vi "DialogCloneMethod.vi"(0 "ClassWriterNative.lvclass":refnum<class "ClassWriterNative.lvclass">, 1 "VIItemRefIn":refnum<vi>, 5 "error in (no error)":errorcluster) -> (11 "NewVIDescriptionOut":string caption="New VI Description", 13 "OpenAfter":bool, 14 "ClassWriterGOOP300.lvclassOut":refnum<class "ClassWriterNative.lvclass">, 15 "VIItemRefOut":refnum<vi>, 16 "NewVIPath":path, 17 "Cancelled":bool, 18 "LibraryOwners":refnum<vi>[](array[refnum]), 19 "error out":errorcluster)   [LabVIEW 2020, in "ClassWriterNative.lvclass"]
uses:
  <resource>/Framework/Providers/Open_GDS/ClassProviders/Provider_LvNativeClass/ClassWriterNative_class/ClassWriterNative.lvclass
  <vilib>/Utility/lvfile.llb/NI_FileType.lvlib
panel:
  in  "Help":bool
  out "ProductPicture":picture
  in  "_NewVIDescription":string caption="New VI Description"
  in  "_CreateOpenVI":bool
  in  "_OverwirteTragetVIs":bool
  in  "_CloneMethodClasses":i32[](listbox) caption="Select which classes to clone the VI to"
  out "_ViPathAlreadyExists":bool=TRUE caption="This VI already exists"
  out "_CloneViName":string caption="Original VI Name"
  in  "_ClassOwner":u16(ring) caption="New VI Owner" items=["<No owner selected>", "<Clone VI to Selected Classes>"]
  in  "_ShowContextHelp":bool
  in  "_NewVIPath":path caption="New VI path"
  in  "_NewVIName":string caption="New VI name"
  in  "_Cancel":bool
  in  "_CloneVI":bool
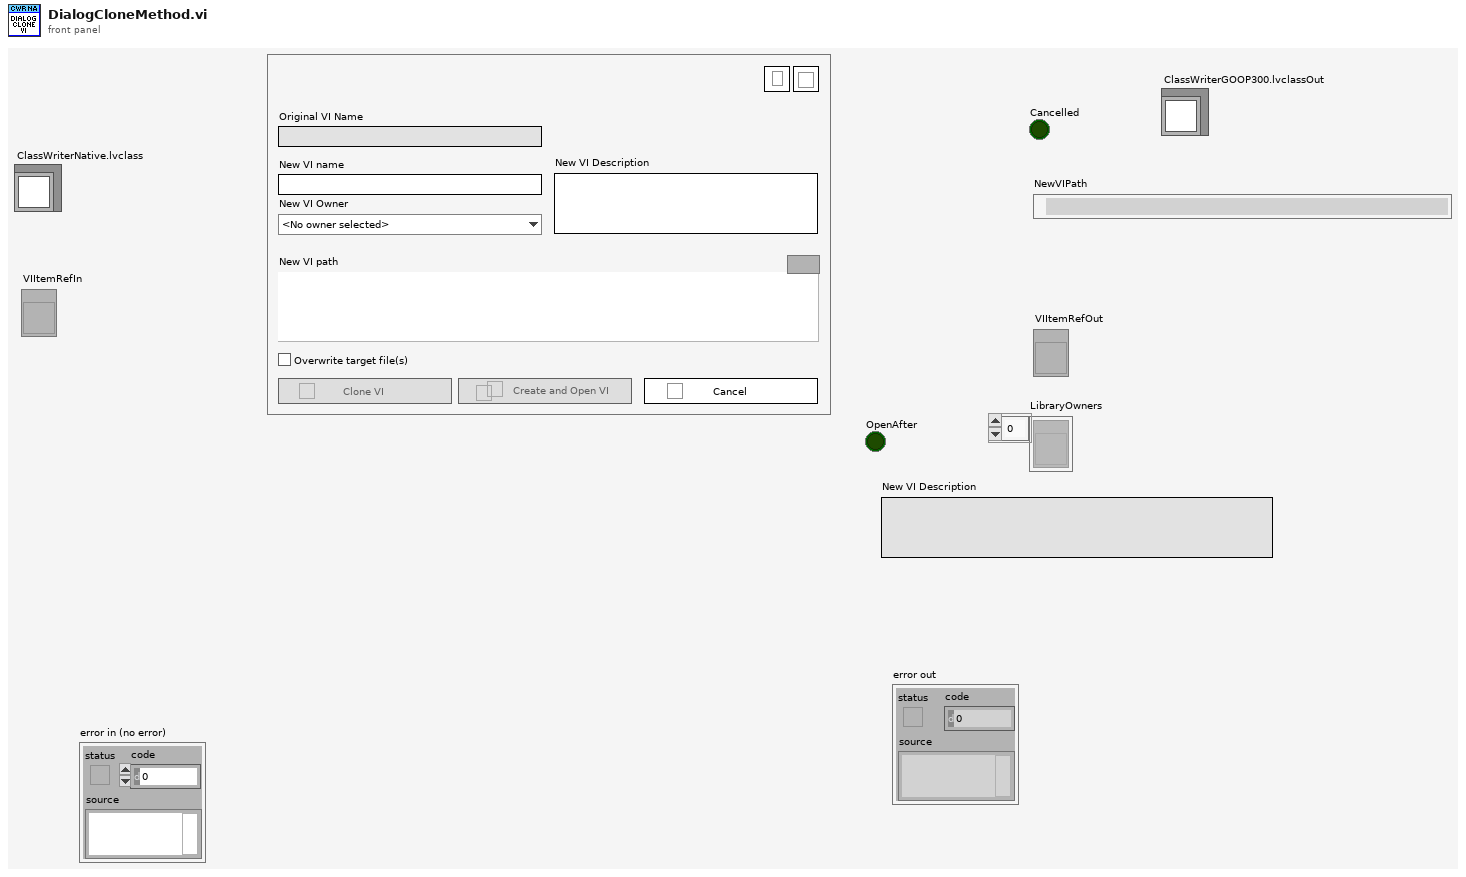
[diagram p1: front panel]
types:
  T1 = cluster{"Cancel":bool, "OrgVIPath":path, "VIName":string, "Libs":refnum<vi>[], "SiblingClasses":refnum<vi>[], "ProjectFolder":path, "ViRelFromParent":path, "VIExt":string, "ManyClasses":bool, "OrgLibName":string, "AllClasses":refnum<vi>[], "OpenAfter":bool}
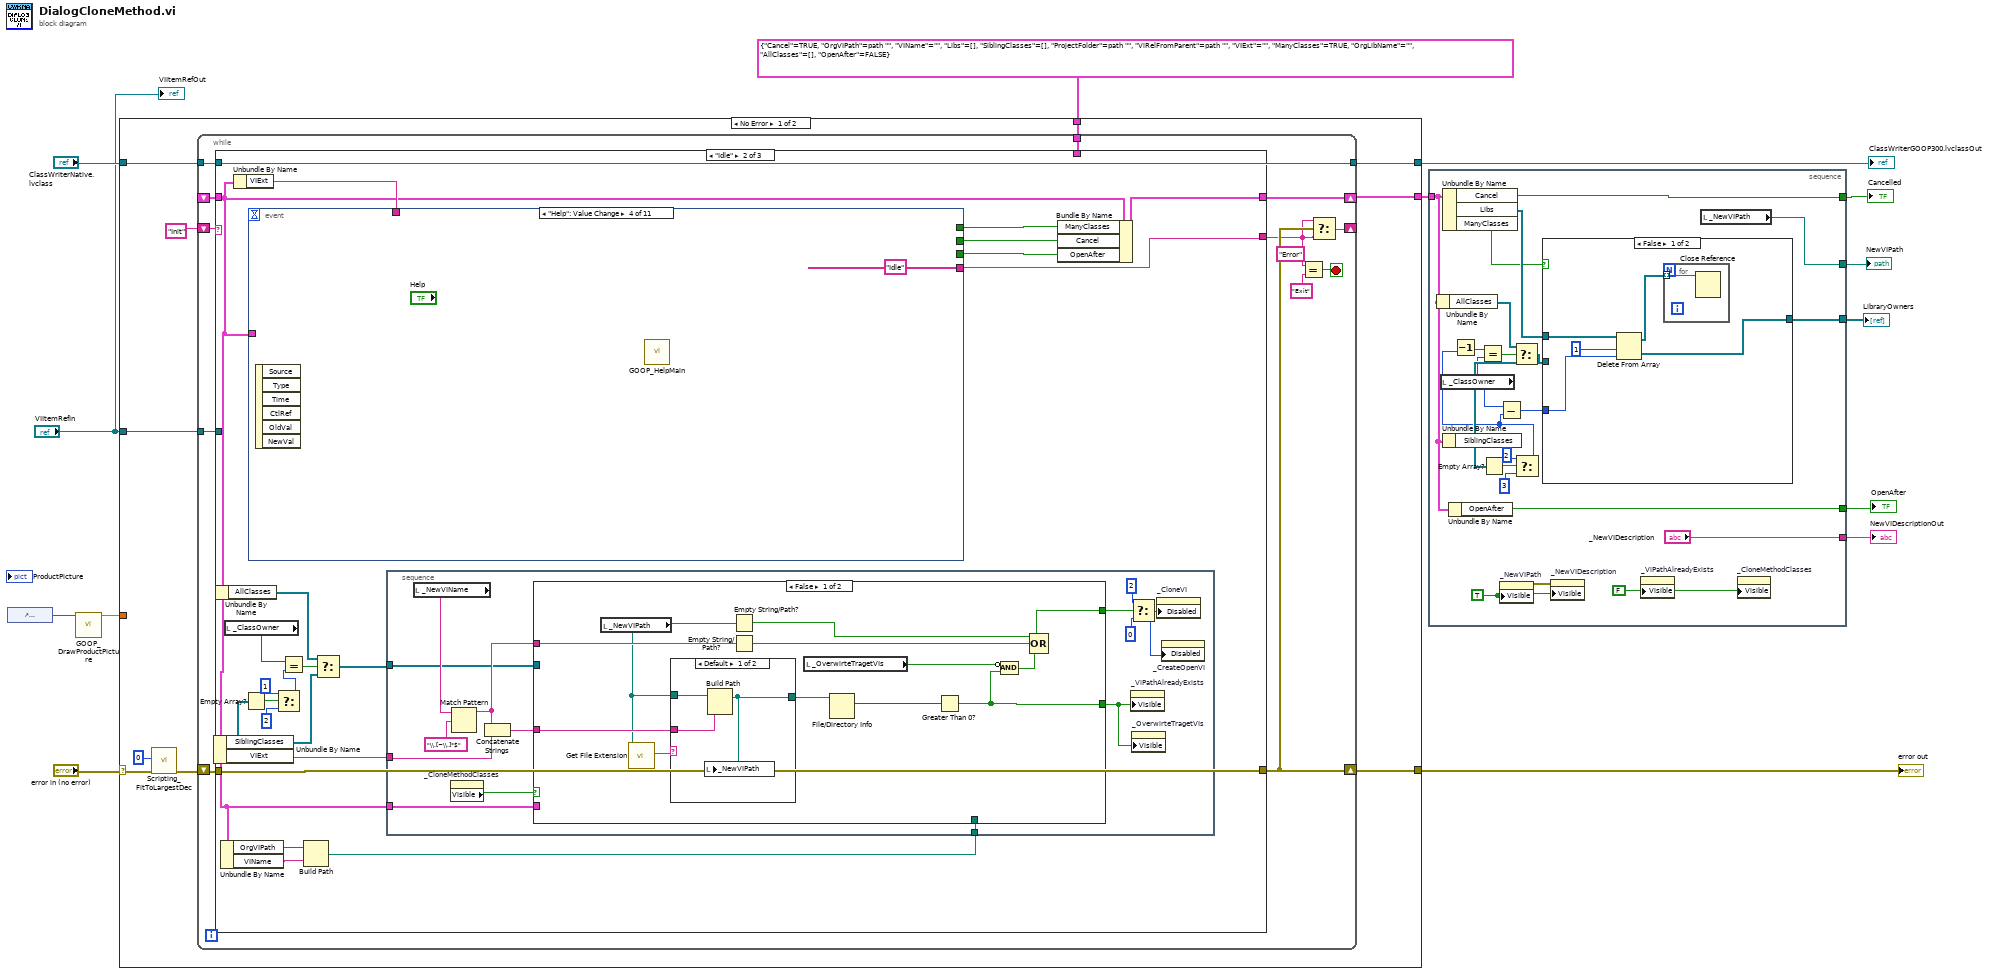
[diagram p0: block diagram]
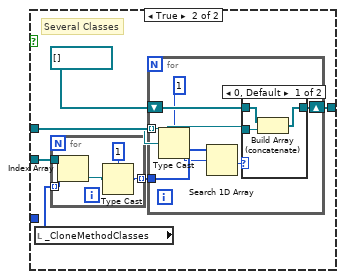
[diagram p2: hidden frame]
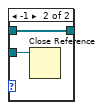
[diagram p3: hidden frame]
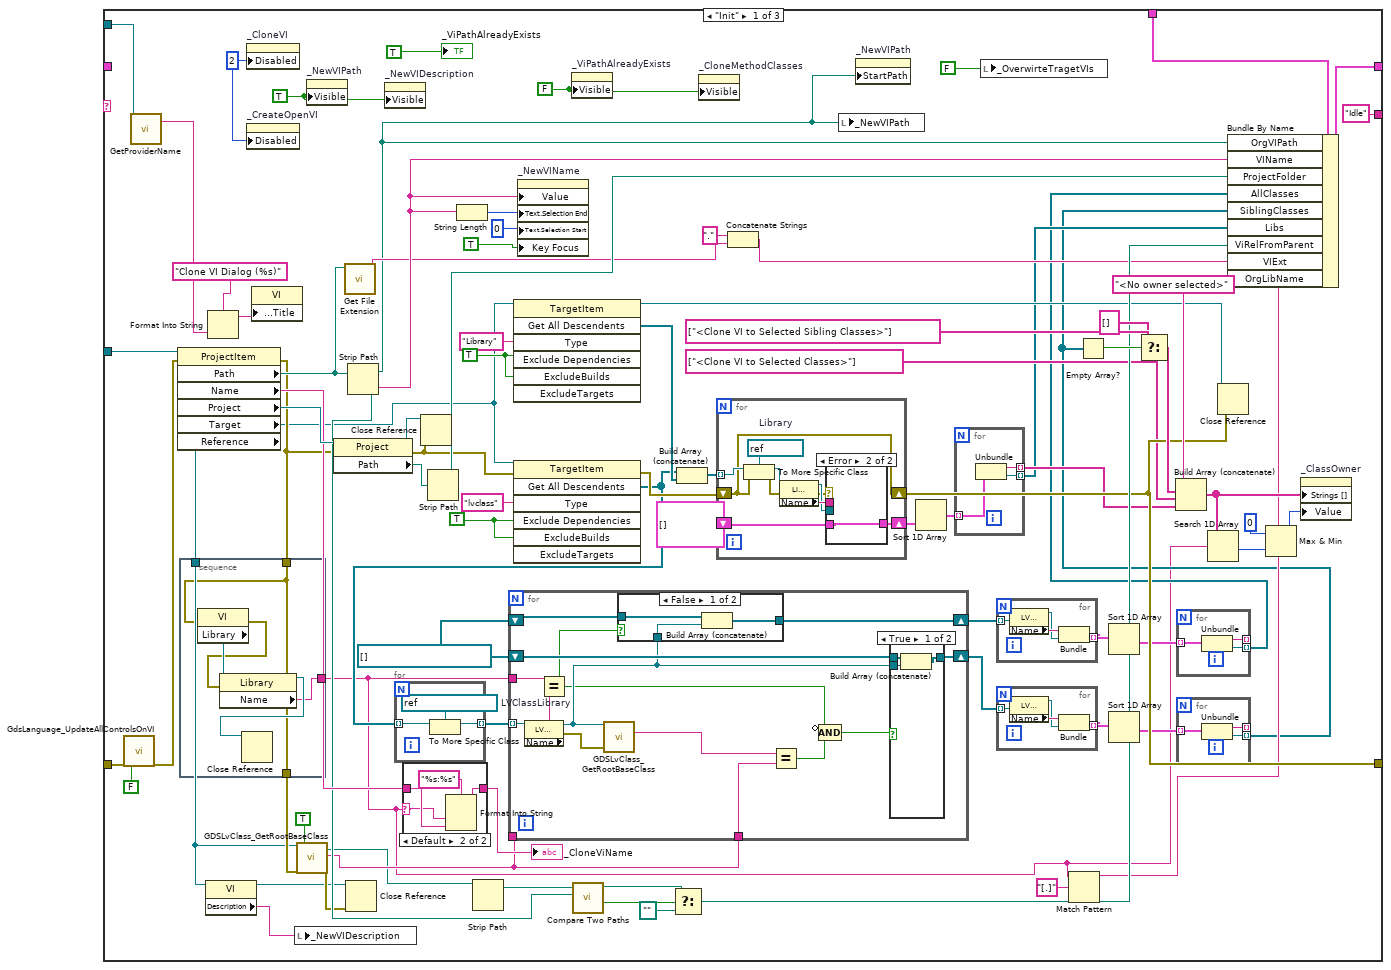
[diagram p4: hidden frame]
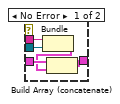
[diagram p8: hidden frame]
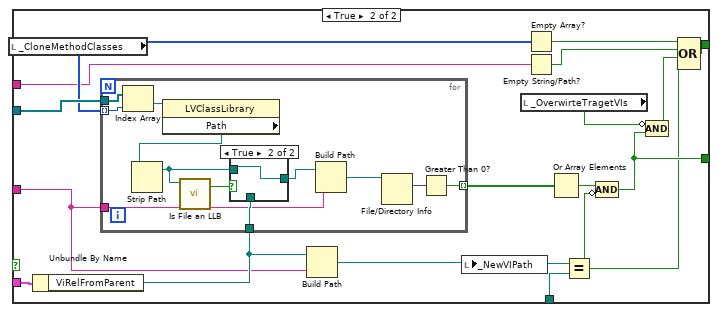
[diagram p10: hidden frame]
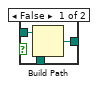
[diagram p11: hidden frame]
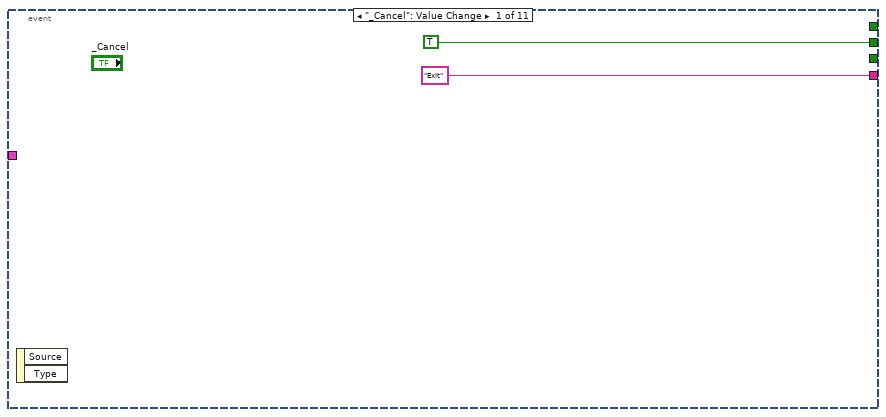
[diagram p12: hidden frame]
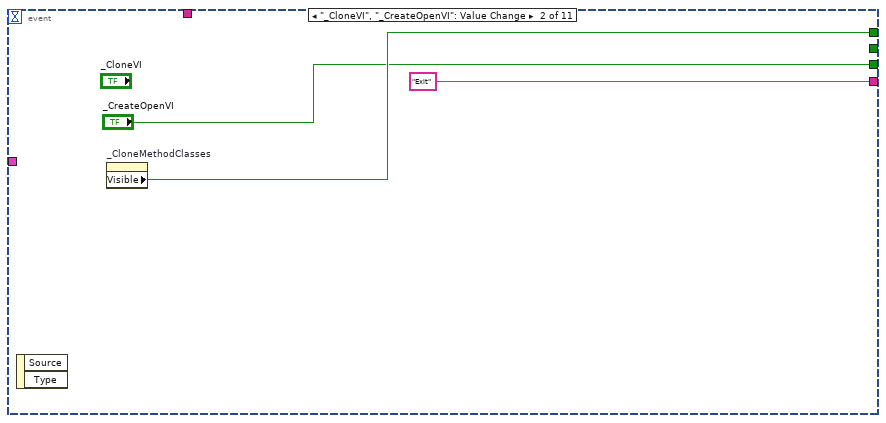
[diagram p13: hidden frame]
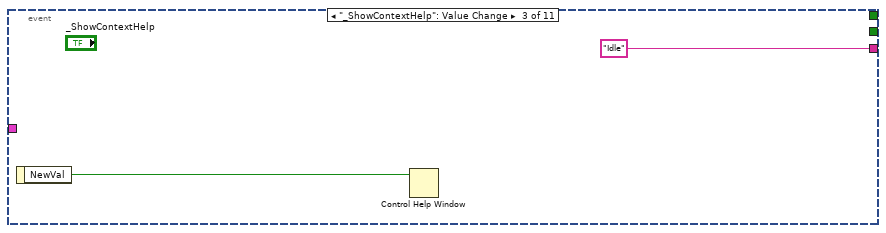
[diagram p14: hidden frame]
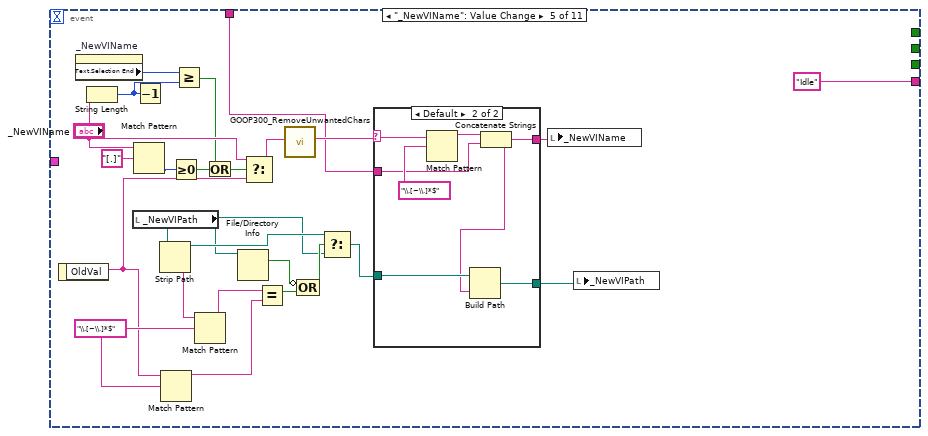
[diagram p15: hidden frame]
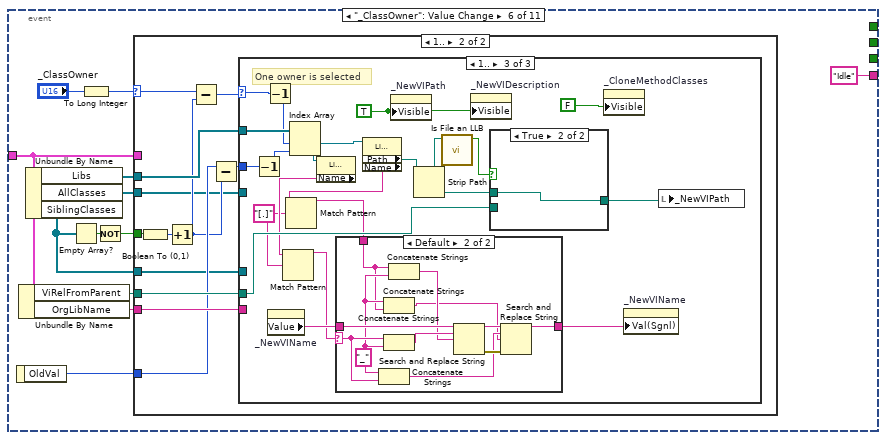
[diagram p17: hidden frame]
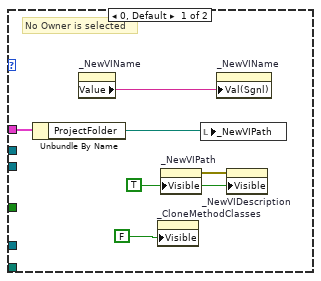
[diagram p18: hidden frame]
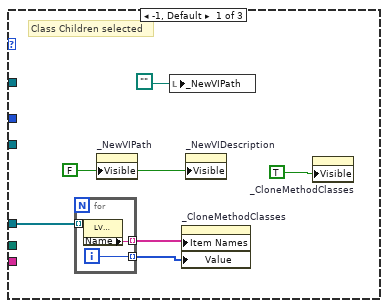
[diagram p19: hidden frame]
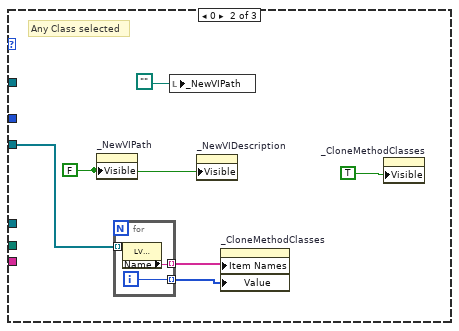
[diagram p20: hidden frame]
diagram:
  n1 = control-ref of="ProductPicture"() -> (w2:refnum<vi>)
  n2 = call <resource>:"GOOP_DrawProductPicture.vi"("ProductPictureControl"=w2) -> ("Zoom Factor"=w1:sgl)  [unwired: 10 in]
  n3 = case shown="No Error" "error in (no error)" {
    selector: "error in (no error)" -> [w17 w419]
    tunnel: "ClassWriterNative.lvclass" -> [w22 w418]
    tunnel: [w24 w419] -> w9
    tunnel: [w23 w418] -> w12
    tunnel: T1 {"Cancel"=TRUE, "OrgVIPath"=path "", "VIName"="", "Libs"=[], "SiblingClasses"=[], "ProjectFolder"=path "", "ViRelFromParent"=path "", "VIExt"="", "ManyClasses"=TRUE, "OrgLibName"="", "AllClasses"=[], "OpenAfter"=FALSE} ("output cluster") -> [w21 _]
    tunnel: "VIItemRefIn" -> [w20 _]
    tunnel: [w19 _] -> w11
    tunnel: w1 -> [_ _]
    frame No Error {
      n4 = call <resource>:"Scripting_FitToLargestDec.vi"("error in (no error)"=w17, "border spacing (2 px)"=0) -> ("error out"=w16:errorcluster)  [unwired: 4 in, 1 out]
      n5 = while {
        shift-right: [w31] -> w24
        shift-left: w16 -> [w37]
        shift-right: [w30] -> _
        shift-left: "Init" -> [w34]
        shift-right: [w35] -> w19
        shift-left: _ -> [w36]
        tunnel: w22 -> [w27]
        tunnel: [w27] -> w23
        tunnel: w21 -> [w26]
        tunnel: w20 -> [w25]
        stop <- w32 stop-if-true
        n6 = case shown="\"Idle\"" w34 {
          tunnel: w36 -> [_ w195 w415]
          tunnel: [w121 w210 w414] -> w35
          tunnel: w37 -> [w111 w212 w416]
          tunnel: [w72 w212 w416] -> w31
          tunnel: w27 -> [w113 _ _]
          tunnel: ["Idle" w211 "Exit"] -> w29
          tunnel: w26 -> [w119 _ _]
          tunnel: w25 -> [w120 _ _]
          frame "Init" {
            w41 = TRUE ("Visible")
            w65 = refnum<vi>[] []
            w97 = TRUE ("ExcludeDependencies")
            w98 = TRUE ("ExcludeDependencies")
            w88 = FALSE ("Visible")
            w63 = u8 2 ("Disabled")
            n7 = call <resource>:"GdsLanguage_UpdateAllControlsOnVI.vi"("error in (no error)"=w111, "CreateLanguageFile(Use this to create a languageFile)"=FALSE) -> ("error out"=w110:errorcluster)  [unwired: 16 in, 1 out]
            n8 = call-dynamic "GetProviderName.vi"("ClassWriterNative in"=w113) -> ("ProviderName"=w112:string)  [unwired: 16 in, 2 out]
            n9 = property class="ProjectItem"(reference=w120, error in=w110) -> (error out=w47:errorcluster, "Path"=w80:path, "Name"=w76:string, "Project"=w107:refnum<vi>, "Target"=w42:refnum<vi>, "Reference"=w40:refnum<vi>)  [unwired: 1 out]
            n10 = stacked-sequence {
              tunnel: w40 -> [w128]
              tunnel: w47 -> [w124]
              tunnel: [w123] -> w45
              tunnel: [w124] -> w46
              frame #0 {
                n11 = property class="VI"(reference=w128, error in=w124) -> (error out=w126:errorcluster, "Library"=w127:refnum<vi>)  [unwired: 1 out]
                n12 = property class="Library"(reference=w127, error in=w126) -> (reference out=w125:refnum<vi>, "Name"=w123:string)  [unwired: 1 out]
                n13 = Close Reference(reference=w125) -> ()  [unwired: 1 in, 1 out]
              }
            }
            n14 = property class="VI"(reference=w40) -> (reference out=w39:refnum<vi>, "Description"=w38:string)  [unwired: 1 in, 1 out]
            n15 = Format Into String(format string="Clone VI Dialog (%s)", w112) -> (resulting string=w115:string)  [unwired: 2 in, 1 out]
            n16 = property on="_CloneVI" class="Bool"("Disabled"=w63) -> ()  [unwired: 2 in, 2 out]
            n17 = property on="_CreateOpenVI" class="Bool"("Disabled"=w63) -> ()  [unwired: 2 in, 2 out]
            n18 = property class="VI"("Front Panel.Title"=w115) -> ()  [unwired: 2 in, 2 out]
            n19 = local write "_NewVIDescription"(w38) -> ()
            n20 = call <resource>:"GDSLvClass_GetRootBaseClass.vi"("ViRef/Path,LvClassRef/Path"=w40, "error in (no error)"=w46, "Don'tOpenReference"=TRUE) -> ("RootBaseClassPath"=w57:path, "ClassName"=w58:string, "error out"=w59:errorcluster)  [unwired: 10 in, 4 out]
            n21 = property on="_NewVIPath" class="Path"("Visible"=w41) -> ()  [unwired: 2 in, 2 out]
            n22 = property class="Project"(reference=w107, error in=w47) -> (reference out=w73:refnum<vi>, error out=w74:errorcluster, "Path"=w81:path)
            n23 = call <vilib>:"Get File Extension.vi"("file"=w80) -> ("lowercase file extension"=w79:string)  [unwired: 6 in, 4 out]
            n24 = Close Reference(reference=w39, error in (no error)=w59) -> ()  [unwired: 1 out]
            n25 = Strip Path(path=w80) -> (stripped path=w70:path, name=w106:string)
            n26 = property on="_NewVIDescription" class="Str"("Visible"=w41) -> ()  [unwired: 2 in, 2 out]
            n27 = case shown="Default" w45 {
              selector: w45 -> [_ w147]
              tunnel: w76 -> [w146 w149]
              tunnel: [w146 w148] -> w75
              frame "" {
              }
              frame Default {
                n28 = Format Into String(format string="%s:%s", w147, w149) -> (resulting string=w148:string)  [unwired: 2 in, 1 out]
              }
            }
            "_CloneViName" <- w75
            n29 = Close Reference(reference=w73, error in (no error)=w74) -> ()  [unwired: 1 out]
            n30 = Strip Path(path=w81) -> (stripped path=w86:path)  [unwired: 1 out]
            n31 = String Length(string=w106) -> (length=w116:i32)
            n32 = Strip Path(path=w57) -> (stripped path=w87:path)  [unwired: 1 out]
            n33 = invoke class="TargetItem" method="Get All Descendents"(reference=w42, "Type"="Library", "Exclude Dependencies"=w98, "ExcludeBuilds"=w98) -> (reference out=w71:refnum<vi>, "All Descendents"=w96:refnum<vi>[])  [unwired: 3 in, 5 out]
            n34 = invoke class="TargetItem" method="Get All Descendents"(reference=w42, error in=w74, "Type"="lvclass", "Exclude Dependencies"=w97, "ExcludeBuilds"=w97) -> (error out=w104:errorcluster, "All Descendents"=w94:refnum<vi>[])  [unwired: 2 in, 5 out]
            n35 = for {
              tunnel: w94 -> [w152] mode=indexing
              tunnel: [w151] -> w64 mode=indexing
              w153 = refnum<vi> refnum  # LVClassLibrary
              n36 = To More Specific Class(target class=w153, reference=w152) -> (specific class reference=w151:refnum<vi>)  [unwired: 1 in, 1 out]
            }
            n37 = for {
              tunnel: w64 -> [w167] mode=indexing
              tunnel: w58 -> [w158]
              shift-right: [w165] -> w49
              shift-left: w65 -> [w166]
              shift-right: [w162] -> w53
              shift-left: w65 -> [w163]
              tunnel: w58 -> [_]
              tunnel: w45 -> [w161]
              n38 = property class="LVClassLibrary"(reference=w167) -> (reference out=w160:refnum<vi>, error out=w159:errorcluster, "Name"=w164:string)  [unwired: 1 in]
              n39 = Equal?(x=w161, y=w164) -> (x = y?=w156:bool)
              n40 = call <resource>:"GDSLvClass_GetRootBaseClass.vi"("ViRef/Path,LvClassRef/Path"=w160, "error in (no error)"=w159) -> ("ClassName"=w157:string)  [unwired: 11 in, 6 out]
              n41 = case shown="False" w156 {
                tunnel: w163 -> [w170 w171]
                tunnel: w160 -> [w169 _]
                tunnel: [w168 w171] -> w162
                frame False {
                  n42 = Build Array (concatenate)(w170, w169) -> (w168:refnum<vi>[])
                }
                frame True {
                }
              }
              n43 = Equal?(x=w157, y=w158) -> (x = y?=w155:bool)
              n44 = Compound Arithmetic op=AND(invert w156, w155) -> (w154:bool)
              n45 = case shown="True" w154 {
                tunnel: w166 -> [w174 w175]
                tunnel: w160 -> [w173 _]
                tunnel: [w172 w175] -> w165
                frame True {
                  n46 = Build Array (concatenate)(w174, w173) -> (w172:refnum<vi>[])
                }
                frame False {
                }
              }
            }
            n47 = property on="_NewVIName" class="Str"("Value"=w106, "Text.Selection End"=w116, "Text.Selection Start"=u32 0 ("Text.Selection:Start"), "Key Focus"=TRUE) -> ()  [unwired: 2 in, 2 out]
            n48 = property on="_ViPathAlreadyExists" class="Bool (strict)"("Visible"=w88) -> ()  [unwired: 2 in, 2 out]
            n49 = call <vilib>:"Compare Two Paths.vi"("Path 2"=w70, "Path 1"=w87) -> ("Path 2 Relative to Path 1?"=w85:bool, "Relative Path from 1 to 2"=w84:path)  [unwired: 6 in, 2 out]
            n50 = Select(t=w84, s=w85, f=path "") -> (s? t:f=w82:path)
            n51 = Build Array (concatenate)(w94, w96) -> (w95:refnum<vi>[])
            n52 = property on="_CloneMethodClasses" class="LstBox (strict)"("Visible"=w88) -> ()  [unwired: 2 in, 2 out]
            n53 = for {
              tunnel: w95 -> [w185] mode=indexing
              shift-right: [w178] -> w72
              shift-left: w104 -> [w178]
              shift-right: [w176] -> w43
              shift-left: cluster{"Name":string, refnum<vi>}[] [] -> [w177]
              w183 = refnum<vi> refnum  # Library
              n54 = To More Specific Class(target class=w183, reference=w185, error in=w178) -> (specific class reference=w184:refnum<vi>, error out=w182:errorcluster)
              n55 = property class="Library"(reference=w184, error in=w182) -> (reference out=w180:refnum<vi>, error out=w179:errorcluster, "Name"=w181:string)
              n56 = case shown="Error" w179 {
                tunnel: w181 -> [w190 _]
                tunnel: w180 -> [w189 _]
                tunnel: w177 -> [w188 w191]
                tunnel: [w186 w191] -> w176
                frame No Error {
                  n57 = Bundle("Name"=w190, w189) -> (w187:cluster{"Name":string, refnum<vi>})  [unwired: 1 in]
                  n58 = Build Array (concatenate)(w188, w187) -> (w186:cluster{"Name":string, refnum<vi>}[])
                }
                frame Error {
                }
              }
            }
            n59 = Concatenate Strings("." ("string"), w79) -> (w78:string)
            n60 = local write "_NewVIPath"(w70) -> ()
            n61 = property on="_NewVIPath" class="Path"("StartPath"=w70) -> ()  [unwired: 2 in, 2 out]
            n62 = Sort 1D Array(array=w43) -> (sorted array=w62:cluster{"Name":string, refnum<vi>}[])
            n63 = for {
              tunnel: w62 -> [w145] mode=indexing
              tunnel: [w144] -> w61 mode=indexing
              tunnel: [w143] -> w60 mode=indexing
              n64 = Unbundle(w145) -> ("Name"=w144:string, w143:refnum<vi>)
            }
            n65 = local write "_OverwirteTragetVIs"(FALSE ("Visible")) -> ()
            n66 = for {
              tunnel: w53 -> [w139] mode=indexing
              tunnel: [w140] -> w55 mode=indexing
              n67 = property class="LVClassLibrary"(reference=w139) -> (reference out=w141:refnum<vi>, "Name"=w142:string)  [unwired: 1 in, 1 out]
              n68 = Bundle("Name"=w142, w141) -> (w140:cluster{"Name":string, refnum<vi>})  [unwired: 1 in]
            }
            n69 = for {
              tunnel: w49 -> [w132] mode=indexing
              tunnel: [w133] -> w50 mode=indexing
              n70 = property class="LVClassLibrary"(reference=w132) -> (reference out=w134:refnum<vi>, "Name"=w135:string)  [unwired: 1 in, 1 out]
              n71 = Bundle("Name"=w135, w134) -> (w133:cluster{"Name":string, refnum<vi>})  [unwired: 1 in]
            }
            n72 = Match Pattern(string=w45, regular expression="[.]") -> (before substring=w68:string)  [unwired: 1 in, 3 out]
            n73 = Sort 1D Array(array=w55) -> (sorted array=w54:cluster{"Name":string, refnum<vi>}[])
            n74 = Sort 1D Array(array=w50) -> (sorted array=w51:cluster{"Name":string, refnum<vi>}[])
            n75 = for {
              tunnel: w54 -> [w138] mode=indexing
              tunnel: [w137] -> _ mode=indexing
              tunnel: [w136] -> w52 mode=indexing
              n76 = Unbundle(w138) -> ("Name"=w137:string, w136:refnum<vi>)
            }
            n77 = for {
              tunnel: w51 -> [w131] mode=indexing
              tunnel: [w130] -> _ mode=indexing
              tunnel: [w129] -> w48 mode=indexing
              n78 = Unbundle(w131) -> ("Name"=w130:string, w129:refnum<vi>)
            }
            n79 = Empty Array?(array=w48) -> (empty?=w92:bool)
            n80 = Select(t=string[] [], s=w92, f=string[] ["<Clone VI to Selected Sibling Classes>"]) -> (s? t:f=w91:string[])
            n81 = Build Array (concatenate)("<No owner selected>", w91, string[] ["<Clone VI to Selected Classes>"], w61) -> (w103:string[])
            n82 = Search 1D Array(1D array=w103, element=w45) -> (index of element=w102:i32)  [unwired: 1 in]
            n83 = Close Reference(reference=w71, error in (no error)=w72) -> ()  [unwired: 1 out]
            n84 = Bundle By Name(cluster=w119, "OrgVIPath"=w70, "VIName"=w106, "ProjectFolder"=w86, "AllClasses"=w52, "SiblingClasses"=w48, "Libs"=w60, "ViRelFromParent"=w82, "VIExt"=w78, "OrgLibName"=w68) -> (w121:T1)
            n85 = Max & Min(x=0 ("Text.Selection:Start"), y=w102) -> (max(x,y)=w100:i32)  [unwired: 1 out]
            n86 = property on="_ClassOwner" class="Ring (strict)"("Strings []"=w103, "Value"=w100) -> ()  [unwired: 2 in, 2 out]
            "_ViPathAlreadyExists" <- TRUE ("Visible")
          }
          frame "Idle" {
            n87 = Unbundle By Name(w195) -> ("SiblingClasses"=w201:refnum<vi>[], "VIExt"=w207:string)
            n88 = Unbundle By Name(w195) -> ("AllClasses"=w204:refnum<vi>[])
            n89 = Unbundle By Name(w195) -> ("OrgVIPath"=w194:path, "VIName"=w193:string)
            n90 = local read "_ClassOwner"() -> (w199:u16)
            n91 = Unbundle By Name(w195) -> ("VIExt"=w208:string)
            n92 = Empty Array?(array=w201) -> (empty?=w202:bool)
            n93 = event shown="[3] \"Help\": Value Change" {
              selector: _ -> [_ _ _ _ _ _ _ _ _ _ _]
              dyn-events: _ -> [_ _ _ _ _ _ _ _ _ _ _]
              timeout: _ -> [_ _ _ _ _ _ _ _ _ _ _]
              tunnel: ["Exit" "Exit" "Idle" "Idle" "Idle" "Idle" "Idle" "Idle" "Idle" "Idle" "Exit"] -> w211
              tunnel: [TRUE _ _ _ _ _ _ _ _ _ w412] -> w209
              tunnel: w195 -> [_ _ _ _ _ w326 _ _ _ _ _]
              tunnel: w208 -> [_ _ _ _ w290 _ _ _ _ _ _]
              tunnel: [_ w279 _ _ _ _ _ _ _ _ _] -> w206
              tunnel: [_ "_CreateOpenVI" _ _ _ _ _ _ _ _ _] -> w196
              event "_Cancel": Value Change {
                n94 = event-data() -> ()  [unwired: 1 in, 2 out]
              }
              event "_CloneVI", "_CreateOpenVI": Value Change {
                n95 = event-data() -> ()  [unwired: 1 in, 2 out]
                n96 = property on="_CloneMethodClasses" class="LstBox (strict)"() -> ("Visible"=w279:bool)  [unwired: 2 in, 2 out]
              }
              event "_ShowContextHelp": Value Change {
                n97 = event-data() -> ("NewVal"=w281:bool)  [unwired: 1 in]
                n98 = Control Help Window(1:w281) -> ()  [unwired: 1 in]
              }
              event "Help": Value Change {
                n99 = event-data() -> ()  [unwired: 1 in, 6 out]
                n100 = call <resource>:"GOOP_HelpMain.vi"() -> ()  [unwired: 12 in]
              }
              event "_NewVIName": Value Change {
                w300 = "\\.[~\\.]*$" ("regular expression")
                n101 = event-data() -> ("OldVal"=w291:string)  [unwired: 1 in]
                n102 = property on="_NewVIName" class="Str"() -> ("Text.Selection End"=w287:u32)  [unwired: 2 in, 2 out]
                n103 = String Length(string="_NewVIName") -> (length=w286:i32)
                n104 = local read "_NewVIPath"() -> (w297:path)
                n105 = Match Pattern(string="_NewVIName", regular expression="[.]") -> (offset past match=w293:i32)  [unwired: 1 in, 3 out]
                n106 = Decrement(x=w286) -> ()  [unwired: 1 out]
                n107 = Strip Path(path=w297) -> (stripped path=w307:path, name=w302:string)
                n108 = Match Pattern(string=w291, regular expression=w300) -> (before substring=w299:string)  [unwired: 1 in, 3 out]
                n109 = Greater Or Equal To 0?(x=w293) -> (x >= 0?=w292:bool)
                n110 = Greater Or Equal?(x=w287, y=w286) -> (x >= y?=w284:bool)
                n111 = Match Pattern(string=w302, regular expression=w300) -> (before substring=w301:string)  [unwired: 1 in, 3 out]
                n112 = Or(x=w284, y=w292) -> (x .or. y?=w285:bool)
                n113 = File/Directory Info(path=w297) -> (directory=w295:bool)  [unwired: 1 in, 6 out]
                n114 = Select(t="_NewVIName", s=w285, f=w291) -> (s? t:f=w289:string)
                n115 = Equal?(x=w301, y=w299) -> (x = y?=w296:bool)
                n116 = call <resource>:"GOOP300_RemoveUnwantedChars.vi"("StringIn"=w289) -> ("StringOut"=w304:string)  [unwired: 10 in]
                n117 = Compound Arithmetic op=OR(invert w295, w296) -> (w298:bool)
                n118 = Select(t=w307, s=w298, f=w297) -> (s? t:f=w306:path)
                n119 = case shown="Default" w304 {
                  selector: w304 -> [w309 w315]
                  tunnel: [w310 w317] -> w305
                  tunnel: w306 -> [w310 w316]
                  tunnel: w290 -> [_ w312]
                  tunnel: [w309 w311] -> w303
                  frame "" {
                  }
                  frame Default {
                    n120 = Match Pattern(string=w315, regular expression="\\.[~\\.]*$") -> (before substring=w313:string)  [unwired: 1 in, 3 out]
                    n121 = Concatenate Strings(w313, w312) -> (w311:string)
                    n122 = Build Path(base path=w316, name or relative path=w311) -> (appended path=w317:path)
                  }
                }
                n123 = local write "_NewVIName"(w303) -> ()
                n124 = local write "_NewVIPath"(w305) -> ()
              }
              event "_ClassOwner": Value Change {
                n125 = event-data() -> ("OldVal"=w321:u16)  [unwired: 1 in]
                n126 = Unbundle By Name(w326) -> ("ViRelFromParent"=w325:path, "OrgLibName"=w322:string)
                n127 = Unbundle By Name(w326) -> ("Libs"=w327:refnum<vi>[], "AllClasses"=w318:refnum<vi>[], "SiblingClasses"=w319:refnum<vi>[])
                n128 = Empty Array?(array=w319) -> (empty?=w328:bool)
                n129 = To Long Integer(number="_ClassOwner") -> (32bit integer=w320:i32)
                n130 = Not(x=w328) -> (.not. x?=w323:bool)
                n131 = case shown="1.." w320 {
                  selector: w320 -> [_ w347]
                  tunnel: w326 -> [w335 _]
                  tunnel: w323 -> [_ w346]
                  tunnel: w327 -> [_ w344]
                  tunnel: w325 -> [_ w343]
                  tunnel: w322 -> [_ w342]
                  tunnel: w321 -> [_ w341]
                  tunnel: w319 -> [_ w337]
                  tunnel: w318 -> [_ w336]
                  frame 0, Default {
                    w330 = TRUE ("Visible")
                    # "No Owner is selected"
                    n132 = Unbundle By Name(w335) -> ("ProjectFolder"=w333:path)
                    n133 = property on="_NewVIName" class="Str"() -> ("Value"=w332:string)  [unwired: 2 in, 2 out]
                    n134 = property on="_CloneMethodClasses" class="LstBox (strict)"("Visible"=FALSE) -> ()  [unwired: 2 in, 2 out]
                    n135 = property on="_NewVIPath" class="Path"("Visible"=w330) -> (error out=w331:errorcluster)  [unwired: 2 in, 1 out]
                    n136 = local write "_NewVIPath"(w333) -> ()
                    n137 = property on="_NewVIName" class="Str"("Val(Sgnl)"=w332) -> ()  [unwired: 2 in, 2 out]
                    n138 = property on="_NewVIDescription" class="Str"(error in=w331, "Visible"=w330) -> ()  [unwired: 1 in, 2 out]
                  }
                  frame 1.. {
                    n139 = Boolean To (0,1)(Boolean=w346) -> (0, 1=w340:i16)
                    n140 = Increment(x=w340) -> (x+1=w338:i16)
                    n141 = Subtract(x=w347, y=w338) -> (x-y=w345:i32)
                    n142 = Subtract(x=w341, y=w338) -> (x-y=w339:u16)
                    n143 = case shown="1.." w345 {
                      selector: w345 -> [_ _ w386]
                      tunnel: w344 -> [_ _ w385]
                      tunnel: w343 -> [_ _ w378]
                      tunnel: w342 -> [_ _ _]
                      tunnel: w339 -> [_ _ w372]
                      tunnel: w337 -> [w351 _ _]
                      tunnel: w336 -> [_ w358 _]
                      frame -1, Default {
                        w348 = FALSE ("Visible")
                        # "Class Children selected"
                        n144 = for {
                          tunnel: [w356] -> w350 mode=indexing
                          tunnel: w351 -> [w355] mode=indexing
                          tunnel: [w354] -> w349 mode=indexing
                          i -> [w354]
                          n145 = property class="LVClassLibrary"(reference=w355) -> ("Name"=w356:string)  [unwired: 1 in, 2 out]
                        }
                        n146 = property on="_NewVIPath" class="Path"("Visible"=w348) -> ()  [unwired: 2 in, 2 out]
                        n147 = local write "_NewVIPath"(path "") -> ()
                        n148 = property on="_CloneMethodClasses" class="LstBox (strict)"("Item Names"=w350, "Value"=w349) -> ()  [unwired: 2 in, 2 out]
                        n149 = property on="_NewVIDescription" class="Str"("Visible"=w348) -> ()  [unwired: 2 in, 2 out]
                        n150 = property on="_CloneMethodClasses" class="LstBox (strict)"("Visible"=TRUE) -> ()  [unwired: 2 in, 2 out]
                      }
                      frame 0 {
                        w357 = FALSE ("Visible")
                        # "Any Class selected"
                        n151 = property on="_NewVIPath" class="Path"("Visible"=w357) -> ()  [unwired: 2 in, 2 out]
                        n152 = for {
                          tunnel: [w365] -> w360 mode=indexing
                          tunnel: w358 -> [w364] mode=indexing
                          tunnel: [w363] -> w359 mode=indexing
                          i -> [w363]
                          n153 = property class="LVClassLibrary"(reference=w364) -> ("Name"=w365:string)  [unwired: 1 in, 2 out]
                        }
                        n154 = local write "_NewVIPath"(path "") -> ()
                        n155 = property on="_NewVIDescription" class="Str"("Visible"=w357) -> ()  [unwired: 2 in, 2 out]
                        n156 = property on="_CloneMethodClasses" class="LstBox (strict)"("Item Names"=w360, "Value"=w359) -> ()  [unwired: 2 in, 2 out]
                        n157 = property on="_CloneMethodClasses" class="LstBox (strict)"("Visible"=TRUE) -> ()  [unwired: 2 in, 2 out]
                      }
                      frame 1.. {
                        w369 = "[.]" ("regular expression")
                        w366 = TRUE ("Visible")
                        # "One owner is selected"
                        n158 = Decrement(x=w372) -> (x-1=w373:u16)
                        n159 = Decrement(x=w386) -> (x-1=w384:i32)
                        n160 = property on="_NewVIName" class="Str"() -> ("Value"=w376:string)  [unwired: 2 in, 2 out]
                        n161 = Index Array(array=w385, index #1=w384, index #2=w373) -> (element #1=w383:refnum<vi>, element #2=w371:refnum<vi>)
                        n162 = property class="Library"(reference=w371) -> ("Name"=w370:string)  [unwired: 1 in, 2 out]
                        n163 = Match Pattern(string=w370, regular expression=w369) -> (before substring=w368:string)  [unwired: 1 in, 3 out]
                        n164 = property class="Library"(reference=w383) -> ("Path"=w381:path, "Name"=w377:string)  [unwired: 1 in, 2 out]
                        n165 = Match Pattern(string=w377, regular expression=w369) -> (before substring=w375:string)  [unwired: 1 in, 3 out]
                        n166 = case shown="Default" w368 {
                          selector: w368 -> [_ w397]
                          tunnel: w376 -> [w387 w398]
                          tunnel: w375 -> [_ w395]
                          tunnel: [w387 w388] -> w374
                          frame "" {
                          }
                          frame Default {
                            w396 = "_" ("string")
                            n167 = Concatenate Strings(w396, w397) -> (w390:string)
                            n168 = Concatenate Strings(w396, w395) -> (w389:string)
                            n169 = Concatenate Strings(w397, w396) -> (w394:string)
                            n170 = Concatenate Strings(w395, w396) -> (w393:string)
                            n171 = Search and Replace String(input string=w398, search string=w394, replace string=w393) -> (result string=w392:string, error out=w391:errorcluster)  [unwired: 5 in, 2 out]
                            n172 = Search and Replace String(input string=w392, search string=w390, replace string=w389, error in=w391) -> (result string=w388:string)  [unwired: 4 in, 3 out]
                          }
                        }
                        n173 = property on="_NewVIPath" class="Path"("Visible"=w366) -> ()  [unwired: 2 in, 2 out]
                        n174 = Strip Path(path=w381) -> (stripped path=w379:path)  [unwired: 1 out]
                        n175 = call <vilib>:"Is File an LLB.vi"("path"=w379) -> ("Is LLB?"=w380:bool)  [unwired: 9 in, 1 out]
                        n176 = property on="_NewVIDescription" class="Str"("Visible"=w366) -> ()  [unwired: 2 in, 2 out]
                        n177 = case shown="True" w380 {
                          tunnel: w379 -> [w401 w402]
                          tunnel: w378 -> [w400 _]
                          tunnel: [w399 w402] -> w382
                          frame False {
                            n178 = Build Path(base path=w401, name or relative path=w400) -> (appended path=w399:path)
                          }
                          frame True {
                          }
                        }
                        n179 = property on="_CloneMethodClasses" class="LstBox (strict)"("Visible"=FALSE) -> ()  [unwired: 2 in, 2 out]
                        n180 = property on="_NewVIName" class="Str"("Val(Sgnl)"=w374) -> ()  [unwired: 2 in, 2 out]
                        n181 = local write "_NewVIPath"(w382) -> ()
                      }
                    }
                  }
                }
              }
              event "_OverwirteTragetVIs": Value Change {
                n182 = event-data() -> ()  [unwired: 1 in, 3 out]
              }
              event "_CloneMethodClasses": Value Change {
                n183 = event-data() -> ()  [unwired: 1 in, 1 out]
              }
              event "_CloneMethodClasses": Shortcut Menu Selection (User) {
                n184 = event-data() -> ()  [unwired: 1 in, 1 out]
                n185 = property on="_CloneMethodClasses" class="LstBox (strict)"() -> ("Item Names"=w405:string[])  [unwired: 2 in, 2 out]
                n186 = for {
                  tunnel: [w408] -> w407 mode=indexing
                  tunnel: w405 -> [_] mode=indexing
                  i -> [w408]
                }
                n187 = local write "_CloneMethodClasses"(w407) -> ()
              }
              event "_NewVIPath": Value Change {
                n188 = event-data() -> ()  [unwired: 1 in, 4 out]
                n189 = property on="_NewVIName" class="Str"() -> ("Value"=w409:string)  [unwired: 2 in, 2 out]
                n190 = property on="_NewVIName" class="Str"("Val(Sgnl)"=w409) -> ()  [unwired: 2 in, 2 out]
              }
              event Panel Close? {
                w412 = TRUE ("Discard?")
                n191 = event-data() -> ()  [unwired: 1 in, 4 out]
                n192 = event-data("Discard?"=w412) -> ()  [unwired: 1 in, 1 out]
              }
            }
            n193 = Select(t=u16 1 ("x"), s=w202, f=u16 2 ("x")) -> (s? t:f=w198:u16)
            n194 = Equal?(x=w199, y=w198) -> (x = y?=w200:bool)
            n195 = Build Path(base path=w194, name or relative path=w193) -> (appended path=w192:path)
            n196 = Select(t=w204, s=w200, f=w201) -> (s? t:f=w205:refnum<vi>[])
            n197 = stacked-sequence {
              tunnel: w207 -> [w220]
              tunnel: w205 -> [w218]
              tunnel: w195 -> [w217]
              tunnel: w192 -> [w213]
              frame #0 {
                n198 = local read "_NewVIName"() -> (w222:string)
                n199 = property on="_CloneMethodClasses" class="LstBox (strict)"() -> ("Visible"=w219:bool)  [unwired: 2 in, 2 out]
                n200 = Match Pattern(string=w222, regular expression="\\.[~\\.]*$") -> (before substring=w221:string)  [unwired: 1 in, 3 out]
                n201 = Concatenate Strings(w221, w220) -> (w224:string)
                n202 = case shown="False" w219 {
                  tunnel: [w238 w255] -> w216
                  tunnel: w224 -> [w237 w253]
                  tunnel: w221 -> [w232 w250]
                  tunnel: [w229 w244] -> w215
                  tunnel: w218 -> [_ w259]
                  tunnel: w217 -> [_ w258]
                  tunnel: w213 -> [_ w246]
                  frame False {
                    n203 = local read "_NewVIPath"() -> (w231:path)
                    n204 = call <vilib>:"Get File Extension.vi"("file"=w231) -> ("lowercase file extension"=w230:string)  [unwired: 6 in, 4 out]
                    n205 = case shown="Default" w230 {
                      tunnel: w237 -> [w241 _]
                      tunnel: [w239 w242] -> w236
                      tunnel: w231 -> [w240 w242]
                      frame Default {
                        n206 = Build Path(base path=w240, name or relative path=w241) -> (appended path=w239:path)
                        n207 = local write "_NewVIPath"(w239) -> ()
                      }
                      frame "ctl", "ctt", "vi", "vit" {
                      }
                    }
                    n208 = Empty String/Path?(string/path=w231) -> (empty?=w233:bool)
                    n209 = Empty String/Path?(string/path=w232) -> (empty?=w234:bool)
                    n210 = local read "_OverwirteTragetVIs"() -> (w227:bool)
                    n211 = File/Directory Info(path=w236) -> (size=w235:i64)  [unwired: 1 in, 6 out]
                    n212 = Greater Than 0?(x=w235) -> (x > 0?=w229:bool)
                    n213 = Compound Arithmetic op=AND(invert w227, w229) -> (w228:bool)
                    n214 = Compound Arithmetic op=OR(w233, w234, w228) -> (w238:bool)
                  }
                  frame True {
                    n215 = local read "_CloneMethodClasses"() -> (w252:i32[])
                    n216 = Unbundle By Name(w258) -> ("ViRelFromParent"=w254:path)
                    n217 = for {
                      tunnel: w259 -> [w271]
                      tunnel: w252 -> [w270] mode=indexing
                      tunnel: w254 -> [w267]
                      tunnel: w253 -> [w265]
                      tunnel: [w262] -> w257 mode=indexing
                      n218 = Index Array(array=w271, index=w270) -> (element=w269:refnum<vi>)
                      n219 = property class="LVClassLibrary"(reference=w269) -> ("Path"=w268:path)  [unwired: 1 in, 2 out]
                      n220 = Strip Path(path=w268) -> (stripped path=w261:path)  [unwired: 1 out]
                      n221 = call <vilib>:"Is File an LLB.vi"("path"=w261) -> ("Is LLB?"=w260:bool)  [unwired: 9 in, 1 out]
                      n222 = case shown="True" w260 {
                        tunnel: w267 -> [w274 _]
                        tunnel: [w273 w275] -> w266
                        tunnel: w261 -> [w272 w275]
                        frame False {
                          n223 = Build Path(base path=w272, name or relative path=w274) -> (appended path=w273:path)
                        }
                        frame True {
                        }
                      }
                      n224 = Build Path(base path=w266, name or relative path=w265) -> (appended path=w263:path)
                      n225 = File/Directory Info(path=w263) -> (size=w264:i64)  [unwired: 1 in, 6 out]
                      n226 = Greater Than 0?(x=w264) -> (x > 0?=w262:bool)
                    }
                    n227 = Build Path(base path=w254, name or relative path=w253) -> (appended path=w247:path)
                    n228 = local write "_NewVIPath"(w247) -> ()
                    n229 = local read "_OverwirteTragetVIs"() -> (w249:bool)
                    n230 = Empty Array?(array=w252) -> (empty?=w251:bool)
                    n231 = Empty String/Path?(string/path=w250) -> (empty?=w256:bool)
                    n232 = Or Array Elements(Boolean array=w257) -> (logical OR=w245:bool)
                    n233 = Equal?(x=w247, y=w246) -> (x = y?=w243:bool)
                    n234 = Compound Arithmetic op=AND(w245, invert w243) -> (w244:bool)
                    n235 = Compound Arithmetic op=AND(invert w249, w244) -> (w248:bool)
                    n236 = Compound Arithmetic op=OR(w251, w256, w248, w243) -> (w255:bool)
                  }
                }
                n237 = Select(t=u8 2, s=w216, f=u8 0 ("Disabled")) -> (s? t:f=w214:u8)
                n238 = property on="_ViPathAlreadyExists" class="Bool (strict)"("Visible"=w215) -> ()  [unwired: 2 in, 2 out]
                n239 = property on="_OverwirteTragetVIs" class="Bool (strict)"("Visible"=w215) -> ()  [unwired: 2 in, 2 out]
                n240 = property on="_CloneVI" class="Bool"("Disabled"=w214) -> ()  [unwired: 2 in, 2 out]
                n241 = property on="_CreateOpenVI" class="Bool"("Disabled"=w214) -> ()  [unwired: 2 in, 2 out]
              }
            }
            n242 = Bundle By Name(cluster=w195, "ManyClasses"=w206, "Cancel"=w209, "OpenAfter"=w196) -> (w210:T1)
          }
          frame "Error", Default {
            n243 = Bundle By Name(cluster=w415, "Cancel"=TRUE) -> (w414:T1)
          }
        }
        n244 = Equal?(x=w29, y="Exit") -> (x = y?=w32:bool)
        n245 = Select(t="Error", s=w31, f=w29) -> (s? t:f=w30:string)
      }
    }
    frame Error {
    }
  }
  "ClassWriterGOOP300.lvclassOut" <- w12
  "error out" <- w9
  n246 = stacked-sequence {
    tunnel: w11 -> [w424]
    tunnel: [w441] -> w10
    tunnel: [w438] -> w6
    tunnel: [w433] -> w5
    tunnel: [w423] -> w4
    tunnel: ["_NewVIDescription"] -> w3
    frame #0 {
      w421 = TRUE ("Visible")
      w440 = FALSE ("Visible")
      n247 = Unbundle By Name(w424) -> ("AllClasses"=w429:refnum<vi>[])
      n248 = local read "_ClassOwner"() -> (w428:u16)
      n249 = Unbundle By Name(w424) -> ("SiblingClasses"=w431:refnum<vi>[])
      n250 = Unbundle By Name(w424) -> ("Cancel"=w441:bool, "Libs"=w439:refnum<vi>[], "ManyClasses"=w432:bool)
      n251 = Unbundle By Name(w424) -> ("OpenAfter"=w423:bool)
      n252 = Empty Array?(array=w431) -> (empty?=w437:bool)
      n253 = property on="_NewVIPath" class="Path"("Visible"=w421) -> (error out=w422:errorcluster)  [unwired: 2 in, 1 out]
      n254 = Select(t=u16 2 ("x"), s=w437, f=u16 3 ("x")) -> (s? t:f=w425:u16)
      n255 = Decrement(x=w425) -> (x-1=w426:u16)
      n256 = Equal?(x=w426, y=w428) -> (x = y?=w427:bool)
      n257 = Subtract(x=w428, y=w425) -> (x-y=w434:u16)
      n258 = Select(t=w429, s=w427, f=w431) -> (s? t:f=w430:refnum<vi>[])
      n259 = case shown="False" w432 {
        tunnel: w439 -> [w446 w453]
        tunnel: [w443 w451] -> w438
        tunnel: w434 -> [w445 _]
        tunnel: w430 -> [_ w450]
        frame False {
          n260 = Delete From Array(array=w446, length=1, index=w445) -> (deleted portion=w443:refnum<vi>[], array with subset deleted=w442:refnum<vi>[])
          n261 = for {
            tunnel: w442 -> [w447] mode=indexing
            n262 = Close Reference(reference=w447) -> ()  [unwired: 1 in, 1 out]
          }
        }
        frame True {
          # "Several Classes"
          n263 = local read "_CloneMethodClasses"() -> (w449:i32[])
          n264 = for {
            tunnel: w450 -> [w458]
            tunnel: w449 -> [w457] mode=indexing
            tunnel: [w455] -> w448 mode=indexing
            n265 = Index Array(array=w458, index=w457) -> (element=w456:refnum<vi>)
            n266 = Type Cast(type=u32 1 ("x"), x=w456) -> (*(type *) &x=w455:u32)
          }
          n267 = for {
            tunnel: w453 -> [w461] mode=indexing
            shift-right: [w464] -> w451
            shift-left: refnum<vi>[] [] -> [w465]
            tunnel: w448 -> [w462]
            n268 = Type Cast(type=u32 1 ("x"), x=w461) -> (*(type *) &x=w459:u32)
            n269 = Search 1D Array(1D array=w462, element=w459) -> (index of element=w463:i32)  [unwired: 1 in]
            n270 = case shown="0, Default" w463 {
              tunnel: w461 -> [w468 w469]
              tunnel: w465 -> [w467 w470]
              tunnel: [w466 w470] -> w464
              frame 0, Default {
                n271 = Build Array (concatenate)(w467, w468) -> (w466:refnum<vi>[])
              }
              frame -1 {
                n272 = Close Reference(reference=w469) -> ()  [unwired: 1 in, 1 out]
              }
            }
          }
        }
      }
      n273 = property on="_NewVIDescription" class="Str"(error in=w422, "Visible"=w421) -> ()  [unwired: 1 in, 2 out]
      n274 = property on="_ViPathAlreadyExists" class="Bool (strict)"("Visible"=w440) -> ()  [unwired: 2 in, 2 out]
      n275 = local read "_NewVIPath"() -> (w433:path)
      n276 = property on="_CloneMethodClasses" class="LstBox (strict)"("Visible"=w440) -> ()  [unwired: 2 in, 2 out]
    }
  }
  "Cancelled" <- w10
  "NewVIPath" <- w5
  "LibraryOwners" <- w6
  "OpenAfter" <- w4
  "NewVIDescriptionOut" <- w3
  "VIItemRefOut" <- "VIItemRefIn"
